vi "I2C_Host_[Top-Level].vi"(4 "CMD_Bytes":u8[](array[numeric])=[48] format="%.0x", 6 "I2C Parameters":T4={"Use_10-Bit_Address"=FALSE, "Slave Device Address"=160, "10-Bit_Address"=0, "NumBytesToRead"=0, "i2c Core Option"=enum."W_To_Device"} {"10-Bit_Address" format="%08b"; "Slave Device Address" format="%08x"}, 7 "Protocol_Timing":T2={"SCL Period (Ticks)"=400, "TransmitDelay(Ticks)"=1000, "PostAddressDelay(Ticks)"=1200, "StartStopDelay(Ticks)"=1200}, 8 "error in (no error)":errorcluster, 11 "I2C Bus":T6) -> (0 "error out":errorcluster, 1 "Status":i16, 2 "FPGA VI Reference Out":T1, 3 "DataBytes":u8[](array[numeric]) caption="Data_Bytes" format="%.0x")   [LabVIEW 2019]
doc: "How to use this VI:\n\n1. Open the I2C Bus by selecting this option in the I2C Bus control & configure the Protocol_Timing parameters and then run the VI. The Protocol_Timing parameters are stored in a un-initialize shift register for the duration of an I2C Bus session. An I2C Bus session starts with Open I2C Bus and ends with Close I2C Bus.\n\nProtocol Timing:\nAll values are in ticks of the 40MHz clock of the FPGA.\nSCL Period = 40MHz / [desired clock rate], for a 100kHz clock use 400 ticks.\nStartStopDelay = number of ticks after or before issuing\nPostAddressDelay = number of ticks after issuing an address on the I2C bus\nTransmitDelay = number of ticks between bytes written, also referred to as InterByteDelay\n\nThe clock, SCL, controls data flow on the SDA so there it is permitted to have delays. These delays are not required but they do help in debugging. The defaults shown are those used during the development process. \n\n2. Once the Bus is Open, meaning the FPGA code has been download and is running with the specified Protocol Timing values, communicating with slave devices is possible. \n\nStart by selecting an option from the i2c Core Option control. After selecting the desired option enter the Slave Device Address, if using a device with a 10-bit address enable the 10-Bit Address Boolean and using the format 1XX011, where XX is the additional address bits, fill in the 10-Bit_Address control. \n\nEnter the command bytes in the CMD_Bytes array in hex.\n\nIf data is to be Read the number of bytes must be specified in NumBytesToRead control. \n\nOnce the desired values have been enter click on the Run button for the VI.\n\nAfter the VI executes the Status is return and if requested, any data bytes in the Data-Byte array.\n\nNote: \nSince the Host VI was designed to be used in a state-machine or in TestStand the CMD_Bytes array can be annoying as it must be cleared from time to time depending on the number of bytes for the command being used. \n\n3. When finished communicating with I2C devices or need to change the Protocol_Timing the I2C Bus must be closed. Select Close I2C Bus from the I2C Bus control and run the VI.\n\n\nStatus Codes\n5001 CMD Timed Out \n5002 Slave Not Responding\n5101 I2C Bus Not Open\n\nWritten By:\nPeter Fuller\nSenior Engineer\nplf Consulting, LLC\nwww.plfconsulting.com\n\nemail: peter@plfconsulting.com\nphone: 617.699.2201"
uses:
  <vilib>/rvi/interface/nirviOpenFPGA/nirviOpenFPGA.xnode
  <vilib>/rvi/interface/nirviReadWriteControl/nirviReadWriteControl.xnode
  <vilib>/rvi/interface/nirviCloseFPGA/nirviCloseFPGA.xnode
  Controls/I2C_Bus_State.ctl
  <vilib>/userDefined/High Color/nirio_resource_hc.ctl
  Controls/FPGA_Reference.ctl
  FPGA Bitfiles/TIsbRIO_FPGATarget_TISensoredBLDC(F_DyXSZt47tvg.lvbitx
  FPGA/TI Sensored BLDC (FPGA).vi
  Controls/Host_I2CBus_Options.ctl
  Controls/i2c_state.ctl
  Controls/i2c_Protocol_Timing.ctl
panel:
  in  "I2C_Bus_State":T5
  # "Internal Controls"
  # "1XX01111"
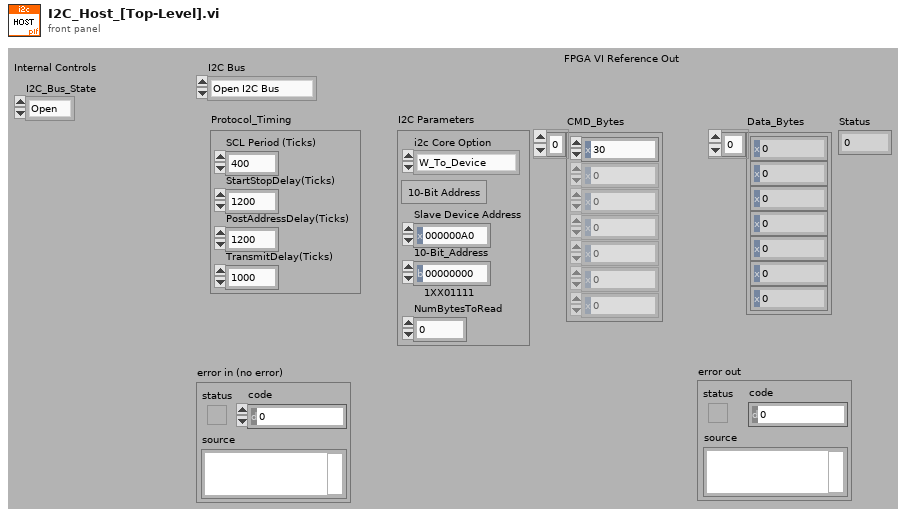
[diagram p1: front panel]
types:
  T1 = typedef "FPGA_Reference.ctl" = refnum<k20>
  T2 = typedef "i2c_Protocol_Timing.ctl" = cluster{"SCL Period (Ticks)":u32, "TransmitDelay(Ticks)":u32, "PostAddressDelay(Ticks)":u32, "StartStopDelay(Ticks)":u32}
  T3 = typedef "i2c_state.ctl" = enum16{"Monitor", "W_To_Device", "R_From_Device", "W/R_From_Device", "TerminateCore"}
  T4 = cluster{"Use_10-Bit_Address":bool, "Slave Device Address":u8, "10-Bit_Address":u8, "NumBytesToRead":i32, "i2c Core Option":T3}
  T5 = typedef "I2C_Bus_State.ctl" = enum16{"Open", "Closed"}
  T6 = typedef "Host_I2CBus_Options.ctl" = enum16{"Open I2C Bus", "Send CMD", "Close I2C Bus"}
  T7 = typedef "nirio_resource_hc.ctl" = tag
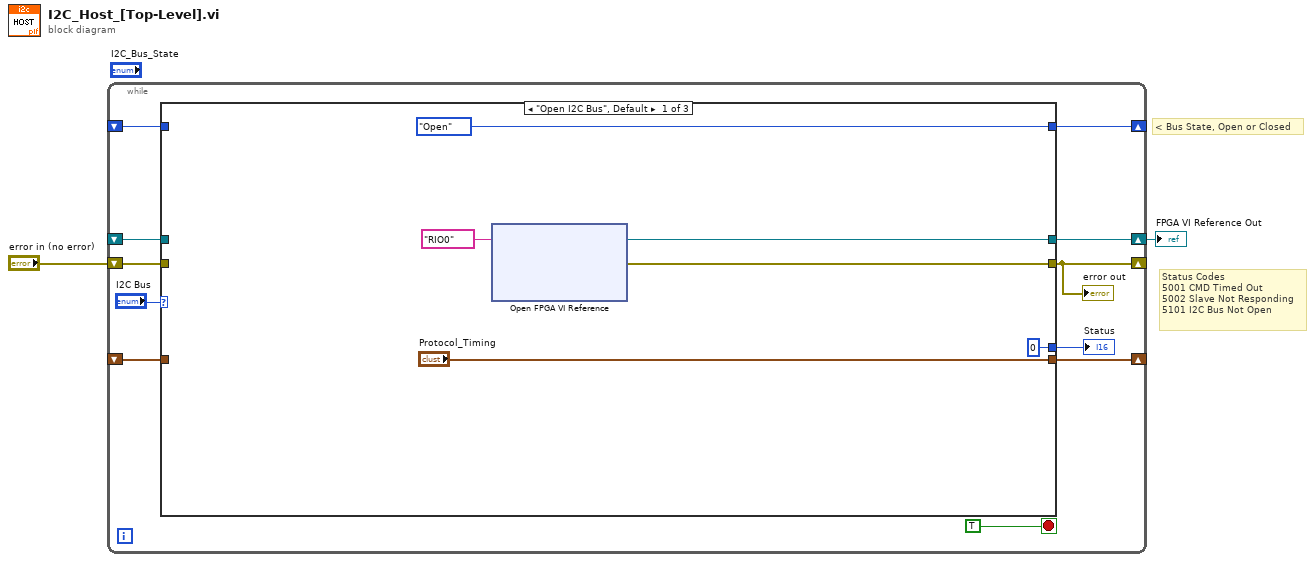
[diagram p0: block diagram]
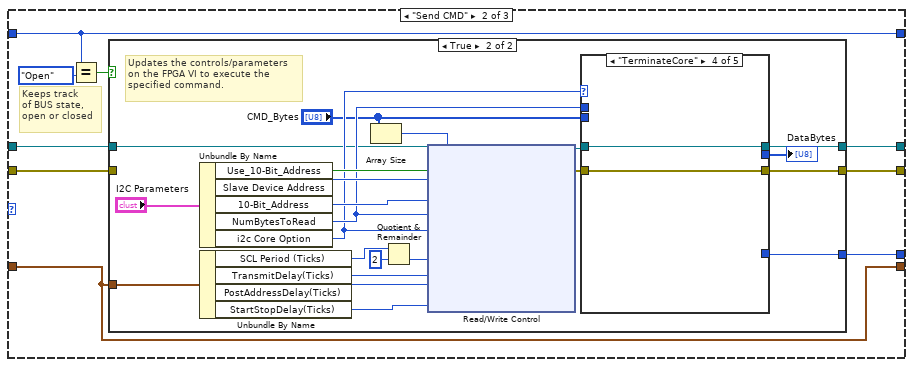
[diagram p2: hidden frame]
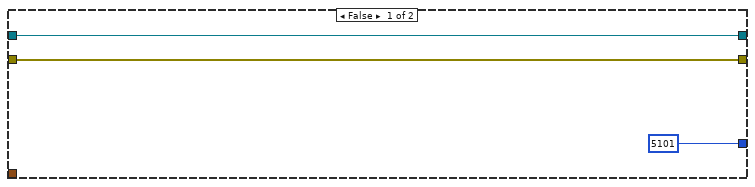
[diagram p3: hidden frame]
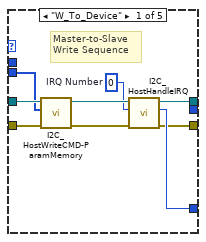
[diagram p4: hidden frame]
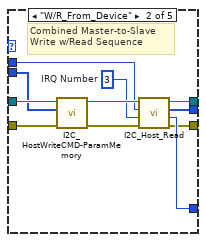
[diagram p5: hidden frame]
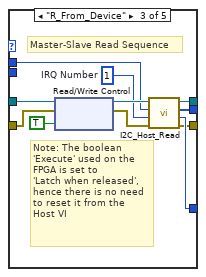
[diagram p6: hidden frame]
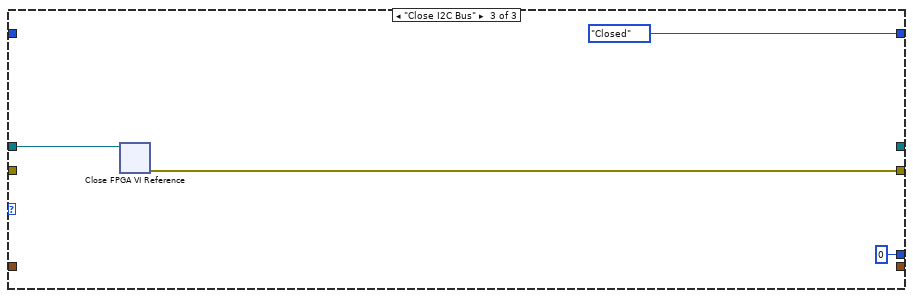
[diagram p8: hidden frame]
diagram:
  # "< Bus State, Open or Closed"
  # "Status Codes\n5001 CMD Timed Out \n5002 Slave Not Responding\n5101 I2C Bus Not Open"
  n1 = while {
    shift-right: [w4] -> w1
    shift-left: _ -> [w13]
    shift-right: [w3] -> _
    shift-left: "error in (no error)" -> [w12]
    shift-right: [w9] -> _
    shift-left: _ -> [w8]
    shift-right: [w7] -> _
    shift-left: _ -> [w6]
    stop <- TRUE stop-if-true
    n2 = case shown="\"Open I2C Bus\", Default" "I2C Bus" {
      tunnel: w13 -> [_ w28 w92]
      tunnel: w12 -> [_ w20 _]
      tunnel: [w14 w27 w91] -> w3
      tunnel: [I2C_Bus_State."Open" ("I2C_Bus_State") w26 I2C_Bus_State."Closed" ("I2C_Bus_State")] -> w9
      tunnel: w8 -> [_ w26 _]
      tunnel: ["Protocol_Timing" w23 _] -> w7
      tunnel: w6 -> [_ w23 _]
      tunnel: [i16 0 ("Status") w22 i16 0 ("Status")] -> w5
      tunnel: [w15 w21 _] -> w4
      frame "Open I2C Bus", Default {
        n3 = xnode "Open FPGA VI Reference"("resource name"=T7 "RIO0") -> ("FPGA VI Reference Out"=w15:T1, "error out"=w14:errorcluster)  [unwired: 1 in]
      }
      frame "Send CMD" {
        # "Keeps track\nof BUS state,\nopen or closed"
        n4 = Equal?(x=w26, y=I2C_Bus_State."Open" ("I2C_Bus_State")) -> (x = y?=w24:bool)
        n5 = case shown="True" w24 {
          tunnel: w28 -> [w30 w33]
          tunnel: w20 -> [w29 _]
          tunnel: [w30 w50] -> w21
          tunnel: [w29 w53] -> w27
          tunnel: [i16 5101 ("Status") w52] -> w22
          tunnel: w23 -> [_ w32]
          frame False {
          }
          frame True {
            # "Updates the controls/parameters\non the FPGA VI to execute the\nspecified command."
            n6 = Unbundle By Name("I2C Parameters") -> ("Use_10-Bit_Address"=w47:bool, "Slave Device Address"=w40:u8, "10-Bit_Address"=w41:u8, "NumBytesToRead"=w37:i32, "i2c Core Option"=w35:T3)
            n7 = Unbundle By Name(w32) -> ("SCL Period (Ticks)"=w44:u32, "TransmitDelay(Ticks)"=w48:u32, "PostAddressDelay(Ticks)"=w45:u32, "StartStopDelay(Ticks)"=w46:u32)
            n8 = Array Size(array="CMD_Bytes") -> (size(s)=w49:i32)
            n9 = Quotient & Remainder(x=w44, y=u32 2) -> (floor(x/y)=w43:u32)  [unwired: 1 out]
            n10 = xnode "Read/Write Control"("FPGA VI Reference In"=w33, "Use_10-Bit_Address"=w47, "Address"=w40, "10-bitAddress"=w41, "NumBytesToRead"=w37, "i2c_State"=w35, "NumBytesToWrite"=w49, "HalfCycle(Ticks)"=w43, "TransmitDelay(Ticks)"=w48, "PostAddressDelay(Ticks)"=w45, "StartStopDelay(Ticks)"=w46) -> ("FPGA VI Reference Out"=w39:T1, "error out"=w38:errorcluster)  [unwired: 1 in]
            n11 = case shown="\"TerminateCore\"" w35 {
              tunnel: [w58 w72 w83 w86 w88] -> w50
              tunnel: [w56 w71 w82 w85 w87] -> w53
              tunnel: [w57 w73 w84 _ _] -> w52
              tunnel: w39 -> [w62 w67 w80 w86 w88]
              tunnel: w38 -> [w60 w66 w77 w85 w87]
              tunnel: "CMD_Bytes" -> [w61 w65 _ _ _]
              tunnel: [_ w68 w81 _ _] -> w51
              tunnel: w37 -> [_ w64 w75 _ _]
              frame "W_To_Device" {
                w54 = 0  # IRQ Number
                # "Master-to-Slave \nWrite Sequence"
                n12 = call "I2C_HostWriteCMD-ParamMemory.vi"("error in"=w60, "CMD-Param_Bytes"=w61, "FPGA VI Reference In"=w62) -> ("error out"=w55:errorcluster, "FPGA VI Reference Out"=w59:T1)  [unwired: 7 out]
                n13 = call "I2C_HostHandleIRQ.vi"("error in"=w55, "IRQ Number"=w54, "FPGA VI Reference In"=w59) -> ("error out"=w56:errorcluster, "Status"=w57:i16, "FPGA VI Reference Out"=w58:T1)  [unwired: 3 in, 3 out]
              }
              frame "W/R_From_Device" {
                w63 = 3  # IRQ Number
                # "Combined Master-to-Slave\nWrite w/Read Sequence"
                n14 = call "I2C_HostWriteCMD-ParamMemory.vi"("error in"=w66, "CMD-Param_Bytes"=w65, "FPGA VI Reference In"=w67) -> ("error out"=w69:errorcluster, "FPGA VI Reference Out"=w70:T1)  [unwired: 7 out]
                n15 = call "I2C_Host_Read.vi"("error in"=w69, "IRQ Number"=w63, "NumBytesToRead"=w64, "FPGA VI Reference In"=w70) -> ("error out"=w71:errorcluster, "Status"=w73:i16, "DataBytes"=w68:u8[], "FPGA VI Reference Out"=w72:T1)  [unwired: 4 out]
              }
              frame "R_From_Device" {
                w74 = 1  # IRQ Number
                # "Note: The boolean\n'Execute' used on the \nFPGA is set to \n'Latch when released', \nhence there is no need\nto reset it from the \nHost VI"
                # "Master-Slave Read Sequence"
                n16 = xnode "Read/Write Control"("FPGA VI Reference In"=w80, "error in"=w77, "Execute"=TRUE) -> ("FPGA VI Reference Out"=w79:T1, "error out"=w78:errorcluster)
                n17 = call "I2C_Host_Read.vi"("error in"=w78, "IRQ Number"=w74, "NumBytesToRead"=w75, "FPGA VI Reference In"=w79) -> ("error out"=w82:errorcluster, "Status"=w84:i16, "DataBytes"=w81:u8[], "FPGA VI Reference Out"=w83:T1)  [unwired: 4 out]
              }
              frame "TerminateCore" {
              }
              frame "Monitor" {
              }
            }
            "DataBytes" <- w51
          }
        }
      }
      frame "Close I2C Bus" {
        n18 = xnode "Close FPGA VI Reference"("FPGA VI Reference In"=w92) -> ("error out"=w91:errorcluster)  [unwired: 1 in]
      }
    }
    "error out" <- w3
    "Status" <- w5
  }
  "FPGA VI Reference Out" <- w1
